vi "find_best_pixel_from_log.vi"(6 "Manual mode?":bool, 7 "Cell details cluster in":T1, 10 "Nth best pixel":i32, 11 "File path of JV log":path) -> (2 "Skip pixel?":bool, 3 "Best pixel cell details cluster":T1)   [LabVIEW 2016]
uses:
  <vilib>/Utility/file.llb/Read From Spreadsheet File (string).vi
panel:
  out "Sorted Array 2":string[][](array[string])
  out "Duplicates removed":string[][](array[string])
  out "Sorted Array":string[][](array[string])
  out "all rows":string[][](array[string])
  out "Nth best pixel 3":i32
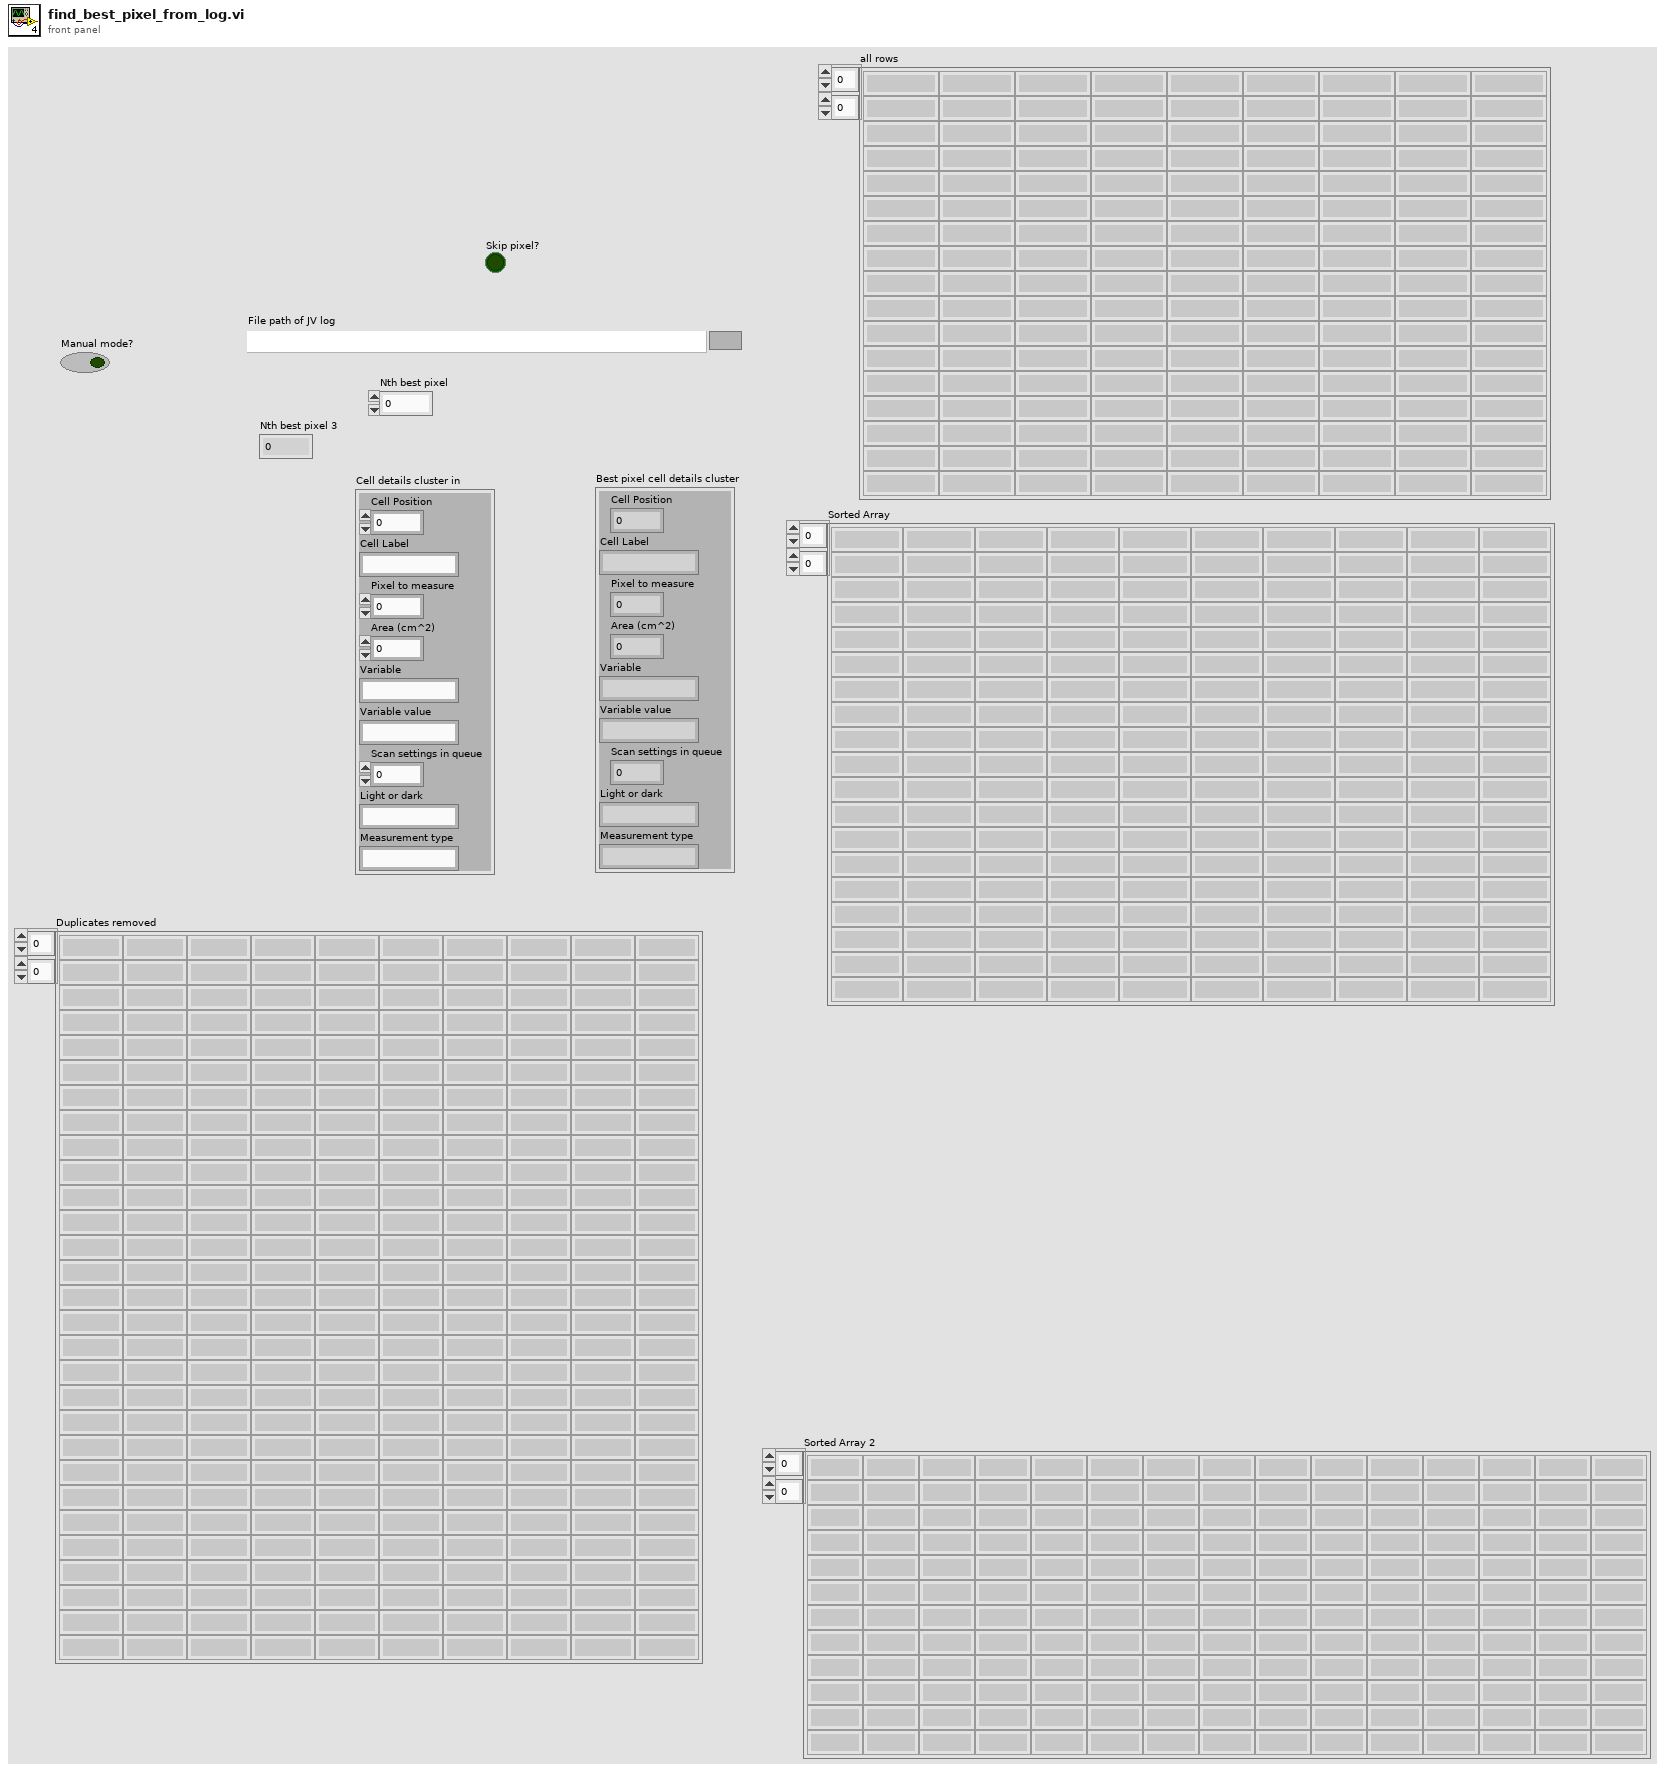
[diagram p1: front panel]
types:
  T1 = cluster{"Cell Position":i32, "Cell Label":string, "Pixel to measure":u16, "Area (cm^2)":dbl, "Variable":string, "Variable value":string, "Scan settings in queue":u16, "Light or dark":string, "Measurement type":string}
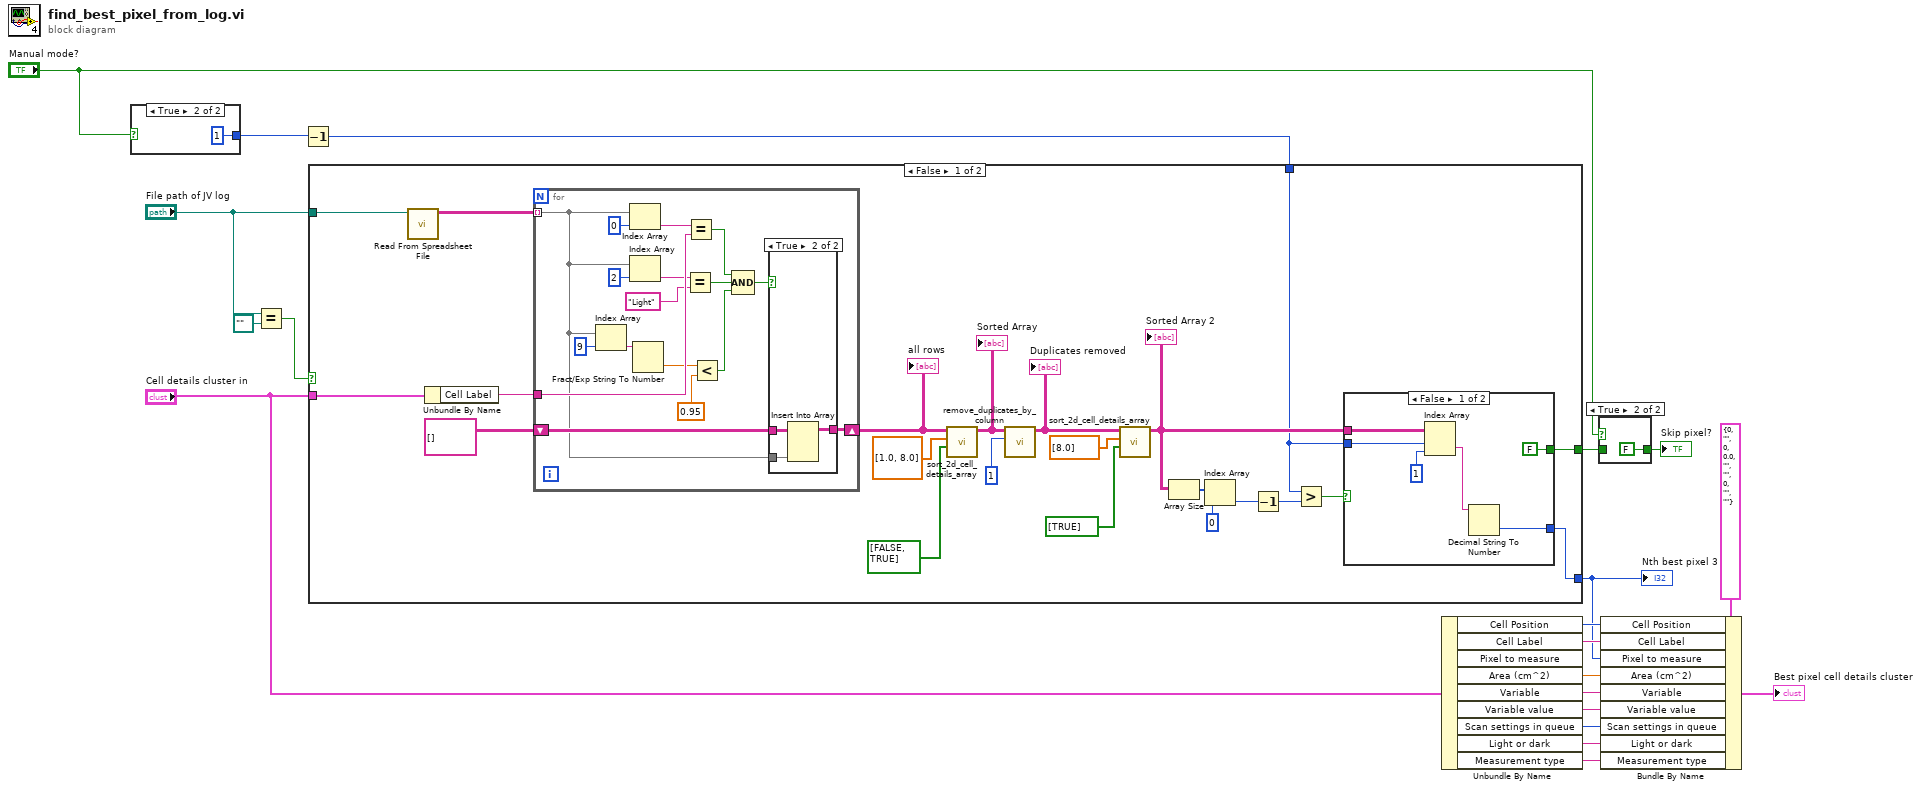
[diagram p0: block diagram]
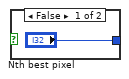
[diagram p3: hidden frame]
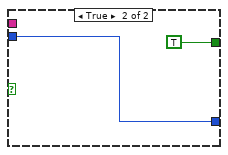
[diagram p4: hidden frame]
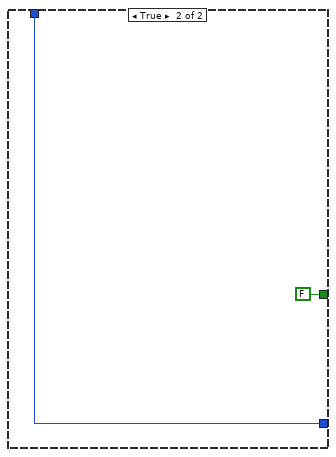
[diagram p6: hidden frame]
diagram:
  n1 = case shown="True" "Manual mode?" {
    tunnel: ["Nth best pixel" 1 ("Nth best pixel")] -> w5
    frame False {
    }
    frame True {
    }
  }
  n2 = Equal?(x="File path of JV log", y=path "") -> (x = y?=w7:bool)
  n3 = Decrement(x=w5) -> (x-1=w4:i32)
  n4 = case shown="False" w7 {
    tunnel: "File path of JV log" -> [w44 _]
    tunnel: [w40 w75] -> w10
    tunnel: w4 -> [w26 w75]
    tunnel: "Cell details cluster in" -> [w32 _]
    tunnel: [w23 FALSE] -> w2
    frame False {
      n5 = call-poly <vilib>:"Read From Spreadsheet File.vi"("file path (dialog if empty)"=w44) -> ("all rows"=w43:string[][])  [unwired: 6 in, 4 out]
      n6 = Unbundle By Name(w32) -> ("Cell Label"=w42:string)
      n7 = for {
        tunnel: w43 -> [w58] mode=indexing
        tunnel: w42 -> [w67]
        shift-right: [w65] -> w39
        shift-left: string[][] [] ("all rows") -> [w66]
        n8 = Index Array(array=w58, index=9) -> (element=w56:string)
        n9 = Index Array(array=w58, index=0) -> (element=w68:string)
        n10 = Index Array(array=w58, index=2) -> (element=w61:string)
        n11 = Fract/Exp String To Number(string=w56) -> (number=w55:dbl)  [unwired: 3 in, 1 out]
        n12 = Equal?(x=w61, y="Light") -> (x = y?=w60:bool)
        n13 = Equal?(x=w68, y=w67) -> (x = y?=w64:bool)
        n14 = Less?(x=w55, y=0.95) -> (x < y?=w53:bool)
        n15 = Compound Arithmetic op=AND(w64, w60, w53) -> (w63:bool)
        n16 = case shown="True" w63 {
          tunnel: w66 -> [w70 w73]
          tunnel: [w70 w72] -> w65
          tunnel: w58 -> [_ w71]
          frame False {
          }
          frame True {
            n17 = Insert Into Array(array=w73, new element=w71) -> (w72:string[][])  [unwired: 2 in]
          }
        }
      }
      "all rows" <- w39
      n18 = call "sort_2d_cell_details_array.vi"("Column descending? array"=bool[] [FALSE, TRUE], "Column priority array"=dbl[] [1.0, 8.0], "Unsorted Array"=w39) -> ("Sorted Array"=w36:string[][])  [unwired: 8 in]
      "Sorted Array" <- w36
      n19 = call "remove_duplicates_by_column.vi"("Column"=1, "Array in"=w36) -> ("Array out"=w31:string[][])  [unwired: 9 in]
      "Duplicates removed" <- w31
      n20 = call "sort_2d_cell_details_array.vi"("Column descending? array"=bool[] [TRUE], "Column priority array"=dbl[] [8.0], "Unsorted Array"=w31) -> ("Sorted Array"=w30:string[][])  [unwired: 8 in]
      "Sorted Array 2" <- w30
      n21 = Array Size(array=w30) -> (size(s)=w29:i32[])
      n22 = Index Array(array=w29, index=0) -> (element=w27:i32)
      n23 = Decrement(x=w27) -> (x-1=w25:i32)
      n24 = Greater?(x=w26, y=w25) -> (0:w24:bool)
      n25 = case shown="False" w24 {
        tunnel: [w50 w52] -> w40
        tunnel: w30 -> [w47 _]
        tunnel: w26 -> [w46 w52]
        tunnel: [FALSE TRUE] -> w23
        frame False {
          n26 = Index Array(array=w47, index (row)=w46, index (col)=1 ("disabled index (col)")) -> (element=w48:string)
          n27 = Decimal String To Number(string=w48) -> (number=w50:i32)  [unwired: 2 in, 1 out]
        }
        frame True {
        }
      }
    }
    frame True {
    }
  }
  "Nth best pixel 3" <- w10
  n28 = Unbundle By Name("Cell details cluster in") -> ("Cell Position"=w19:i32, "Cell Label"=w18:string, "Area (cm^2)"=w16:dbl, "Variable"=w15:string, "Variable value"=w14:string, "Scan settings in queue"=w13:u16, "Light or dark"=w12:string, "Measurement type"=w11:string)  [unwired: 1 out]
  n29 = case shown="True" "Manual mode?" {
    tunnel: [w76 FALSE] -> w3
    tunnel: w2 -> [w76 _]
    frame False {
    }
    frame True {
    }
  }
  "Skip pixel?" <- w3
  n30 = Bundle By Name(cluster=T1 {"Cell Position"=0, "Cell Label"="", "Pixel to measure"=0, "Area (cm^2)"=0.0, "Variable"="", "Variable value"="", "Scan settings in queue"=0, "Light or dark"="", "Measurement type"=""} ("Cell details cluster in"), "Cell Position"=w19, "Cell Label"=w18, "Pixel to measure"=w10, "Area (cm^2)"=w16, "Variable"=w15, "Variable value"=w14, "Scan settings in queue"=w13, "Light or dark"=w12, "Measurement type"=w11) -> (→"Best pixel cell details cluster":T1)
